vi "PPS_TRAJECTORY_CMD_FOLLOW_SWERVE.vi"(6 "Pass_Through_Time":dbl=-1.0 format="%33.4f", 8 "Init":bool) -> (0 "AtReference":bool, 1 "Complete":bool, 3 "Chassis Velocity Target SI":T1 {"vOmega" format="%10.3f"; "vY" format="%10.3f"; "vX" format="%10.3f"})   [LabVIEW 2019]
uses:
  <vilib>/Rock Robotics/WPI/ThirdParty/JAS_Junk/TrajLib/TypeDef/CHASSIS_SPEEDS.ctl
  <vilib>/Rock Robotics/WPI/ThirdParty/JAS_Junk/TrajLib/VI/Util_GetTime_U32.vi
  <vilib>/Rock Robotics/WPI/ThirdParty/JAS_Junk/TrajLib/ProfiledPIDController_NewPeriod.vi
  <vilib>/Rock Robotics/WPI/ThirdParty/JAS_Junk/TrajLib/ProfiledPIDController_SetIntegratorRange.vi
  <vilib>/Rock Robotics/WPI/ThirdParty/JAS_Junk/TrajLib/ProfiledPIDController_DisableContInput.vi
  <vilib>/Rock Robotics/WPI/ThirdParty/JAS_Junk/TrajLib/ProfiledPIDController_EnableContInput.vi
  <vilib>/Rock Robotics/WPI/ThirdParty/JAS_Junk/TrajLib/TrapProfConstraint_New.vi
  <vilib>/Rock Robotics/WPI/ThirdParty/JAS_Junk/TrajLib/Pose2d_New.vi
  <vilib>/Rock Robotics/WPI/ThirdParty/JAS_Junk/TrajLib/Conv_Deg_Radians.vi
  <vilib>/Rock Robotics/WPI/ThirdParty/JAS_Junk/TrajLib/TrapProfState_New.vi
  <vilib>/Rock Robotics/WPI/ThirdParty/JAS_Junk/TrajLib/PIDController_NewPeriod.vi
  <vilib>/Rock Robotics/SystemInterfaces/NetworkCommunication/NetComm_UsageReport_report.vi
  <vilib>/Rock Robotics/WPI/ThirdParty/JAS_Junk/TrajLib/PIDController_SetIntegratorRange.vi
  <vilib>/Rock Robotics/WPI/ThirdParty/JAS_Junk/TrajLib/PIDController_DisableContinousInput.vi
  <vilib>/Rock Robotics/WPI/ThirdParty/JAS_Junk/TrajLib/PIDController_EnableContinousInput.vi
  <vilib>/Rock Robotics/WPI/ThirdParty/JAS_Junk/TrajLib/Rotation2d_CreateAngle.vi
  <vilib>/Rock Robotics/WPI/ThirdParty/JAS_Junk/TrajLib/Translation2d_Create.vi
  PPS_TRAJECTORY_GLOBALS.vi
  Swerve_Drive_System/PPS_DRIVE_GLOBALS.vi
  <vilib>/Rock Robotics/WPI/ThirdParty/JAS_Junk/TrajLib/Globals/Util_LibraryGlobals.vi
  <vilib>/Rock Robotics/WPI/ThirdParty/JAS_Junk/TrajLib/VI/Util_GetTime_U64.vi
  <vilib>/Rock Robotics/WPI/ThirdParty/JAS_Junk/TrajLib/Trajectory_Library.lvlib
  <vilib>/Rock Robotics/WPI/ThirdParty/MJansen/PathPlanner/PathPlanner24.lvlib
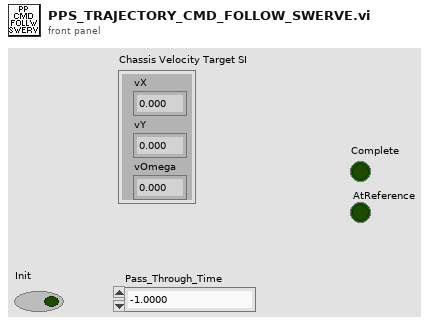
[diagram p1: front panel]
types:
  T1 = typedef "Trajectory_Library.lvlib/CHASSIS_SPEEDS.ctl" = cluster{"vX":dbl, "vY":dbl, "vOmega":dbl}
  T2 = typedef "PathPlanner24.lvlib/PathPlannerPath.ctl" = cluster{"BezierPoints":T3[], "PreviewStartingRotation":T4, "Reversed":bool, "RotationTargets":T5[], "ConstraintZones":T6[], "EventMarkers":T8[], "GlobalConstraints":T7, "GoalEndState":T11, "AllPoints":T12[]}
  T3 = typedef "Trajectory_Library.lvlib/TRANSLATION2D.ctl" = cluster{"X":dbl, "Y":dbl}
  T4 = typedef "Trajectory_Library.lvlib/ROTATION2D.ctl" = cluster{"VALUE":dbl, "COS":dbl, "SIN":dbl}
  T5 = typedef "PathPlanner24.lvlib/PathPlannerRotationTarget.ctl" = cluster{"target":T4, "WaypointRelativePosition":dbl, "Exists":bool}
  T6 = typedef "PathPlanner24.lvlib/PathPlannerConstraintsZone.ctl" = cluster{"minWaypointPos":dbl, "maxWaypointPos":dbl, "Constraints":T7, "Present":bool}
  T7 = typedef "PathPlanner24.lvlib/PathPlannerPathConstraints.ctl" = cluster{"MaxVelocityMps;":dbl, "MaxAccelerationMpsSq;":dbl, "MaxAngularVelRadPsEc;":dbl, "MaxAngularAccRadPSecSq":dbl, "Exists":bool}
  T8 = typedef "PathPlanner24.lvlib/PathPlannerEventMarker.ctl" = cluster{"WaypointRelativePos":dbl, "minimumTriggerDistance":dbl, "markerPos":T3, "lastRobotPos":T3, "Command":T9, "markerPos Exists":bool, "LastRobotPoseExists":bool, "Triggered":bool}
  T9 = typedef "PathPlanner24.lvlib/PathPlannerCommandUtil.ctl" = cluster{"waitTime":dbl, "name":string, "pathName":string, "commands":cluster{"type":T10, "waitTime":dbl, "name":string, "pathName":string}[], "type":T10}
  T10 = typedef "PathPlanner24.lvlib/PathPlanner_CommandUtilType_ENUM.ctl" = enum16{"Unknown", "Wait", "Named", "Path", "Sequential", "Parallel", "Race", "Deadline"}
  T11 = typedef "PathPlanner24.lvlib/PathPlannerGoalEndState.ctl" = cluster{"Velocity":dbl, "Rotation":T4}
  T12 = typedef "PathPlanner24.lvlib/PathPlannerPathPoint.ctl" = cluster{"Position":T3, "HolonomicRotation":T4, "DistAlongPath":dbl, "CurveRadius":dbl, "MaxV":dbl, "Constraints":T7, "HolonomicRotationExists":bool}
  T13 = typedef "Trajectory_Library.lvlib/PID_TUNING.ctl" = cluster{"Kp":dbl, "Ki":dbl, "Kd":dbl, "MaximumIntegral":dbl, "MinimumIntegral":dbl}
  T14 = typedef "Trajectory_Library.lvlib/POSE2D.ctl" = cluster{"TRANSLATION":T3, "ROTATION":T4}
  T15 = typedef "Trajectory_Library.lvlib/PROFILED_PID_CONTROLLER.ctl" = cluster{"Controller":T16, "Goal":T17, "Setpoint":T17, "Constraint":T18}
  T16 = typedef "Trajectory_Library.lvlib/PID_CONTROLLER.ctl" = cluster{"Kp":dbl, "Ki":dbl, "Kd":dbl, "Period":dbl, "Max_Integral":dbl, "Min_Integral":dbl, "Max_Input":dbl, "Min_Input":dbl, "Continuous":bool, "PositionError":dbl, "VelocityError":dbl, "PrevError":dbl, "TotalError":dbl, "PositionTolerance":dbl, "VelocityTolerance":dbl, "SetPoint":dbl, "Kf":dbl, "Prev_Deriv":dbl, "Prev_Deriv 2":dbl, "DerivativeFilter":bool, "Min_Output":dbl, "Max_Output":dbl, "Prev_F_P":dbl, "Prev_F_P_2":dbl, "AntiWindupActive":bool, "Measurement":dbl}
  T17 = typedef "Trajectory_Library.lvlib/TRAPEZOID_PROFILE_STATE.ctl" = cluster{"Position":dbl, "Velocity":dbl}
  T18 = typedef "Trajectory_Library.lvlib/TRAPEZOID_PROFILE_CONSTRAINT.ctl" = cluster{"MaxVelocity":dbl, "MaxAcceleration":dbl}
  T19 = typedef "PathPlanner24.lvlib/PathPlannerReplanningConfig.ctl" = cluster{"enableInitialReplanning":bool, "enableDynamicReplanning":bool, "dynamicReplanningTotalErrorThreshold":dbl, "dynamicReplanningErrorSpikeThreshold":dbl}
  T20 = typedef "Trajectory_Library.lvlib/HOLONOMIC_PACK_TUNING.ctl" = cluster{"X PID Tuning":T13, "Y PID Tuning":T13, "thetaProfiledPID_CTRL":T15}
  T21 = typedef "PathPlanner24.lvlib/PathPlannerCmdFollowHolConfig.ctl" = cluster{"HOLONOMIC_CTRL_PACK_TUNING":T20, "Max Wheel Speed M/S":dbl, "Tolerance SI":T14, "Drive Base Radius M":dbl, "ControlPastEnd_Sec":dbl, "ReplanningConfig":T19, "Period_Sec":dbl, "Trigger Events":bool}
  T22 = typedef "Trajectory_Library.lvlib/HOLONOMIC_DRV_CTRL.ctl" = cluster{"poseTolerance":T14, "poseError":T14, "Enabled":bool, "PID_xCtrl":T16, "PID_yCtrl":T16, "PROF_PID_thetaCtrl":T15, "RotationError":T4, "FirstRun":bool}
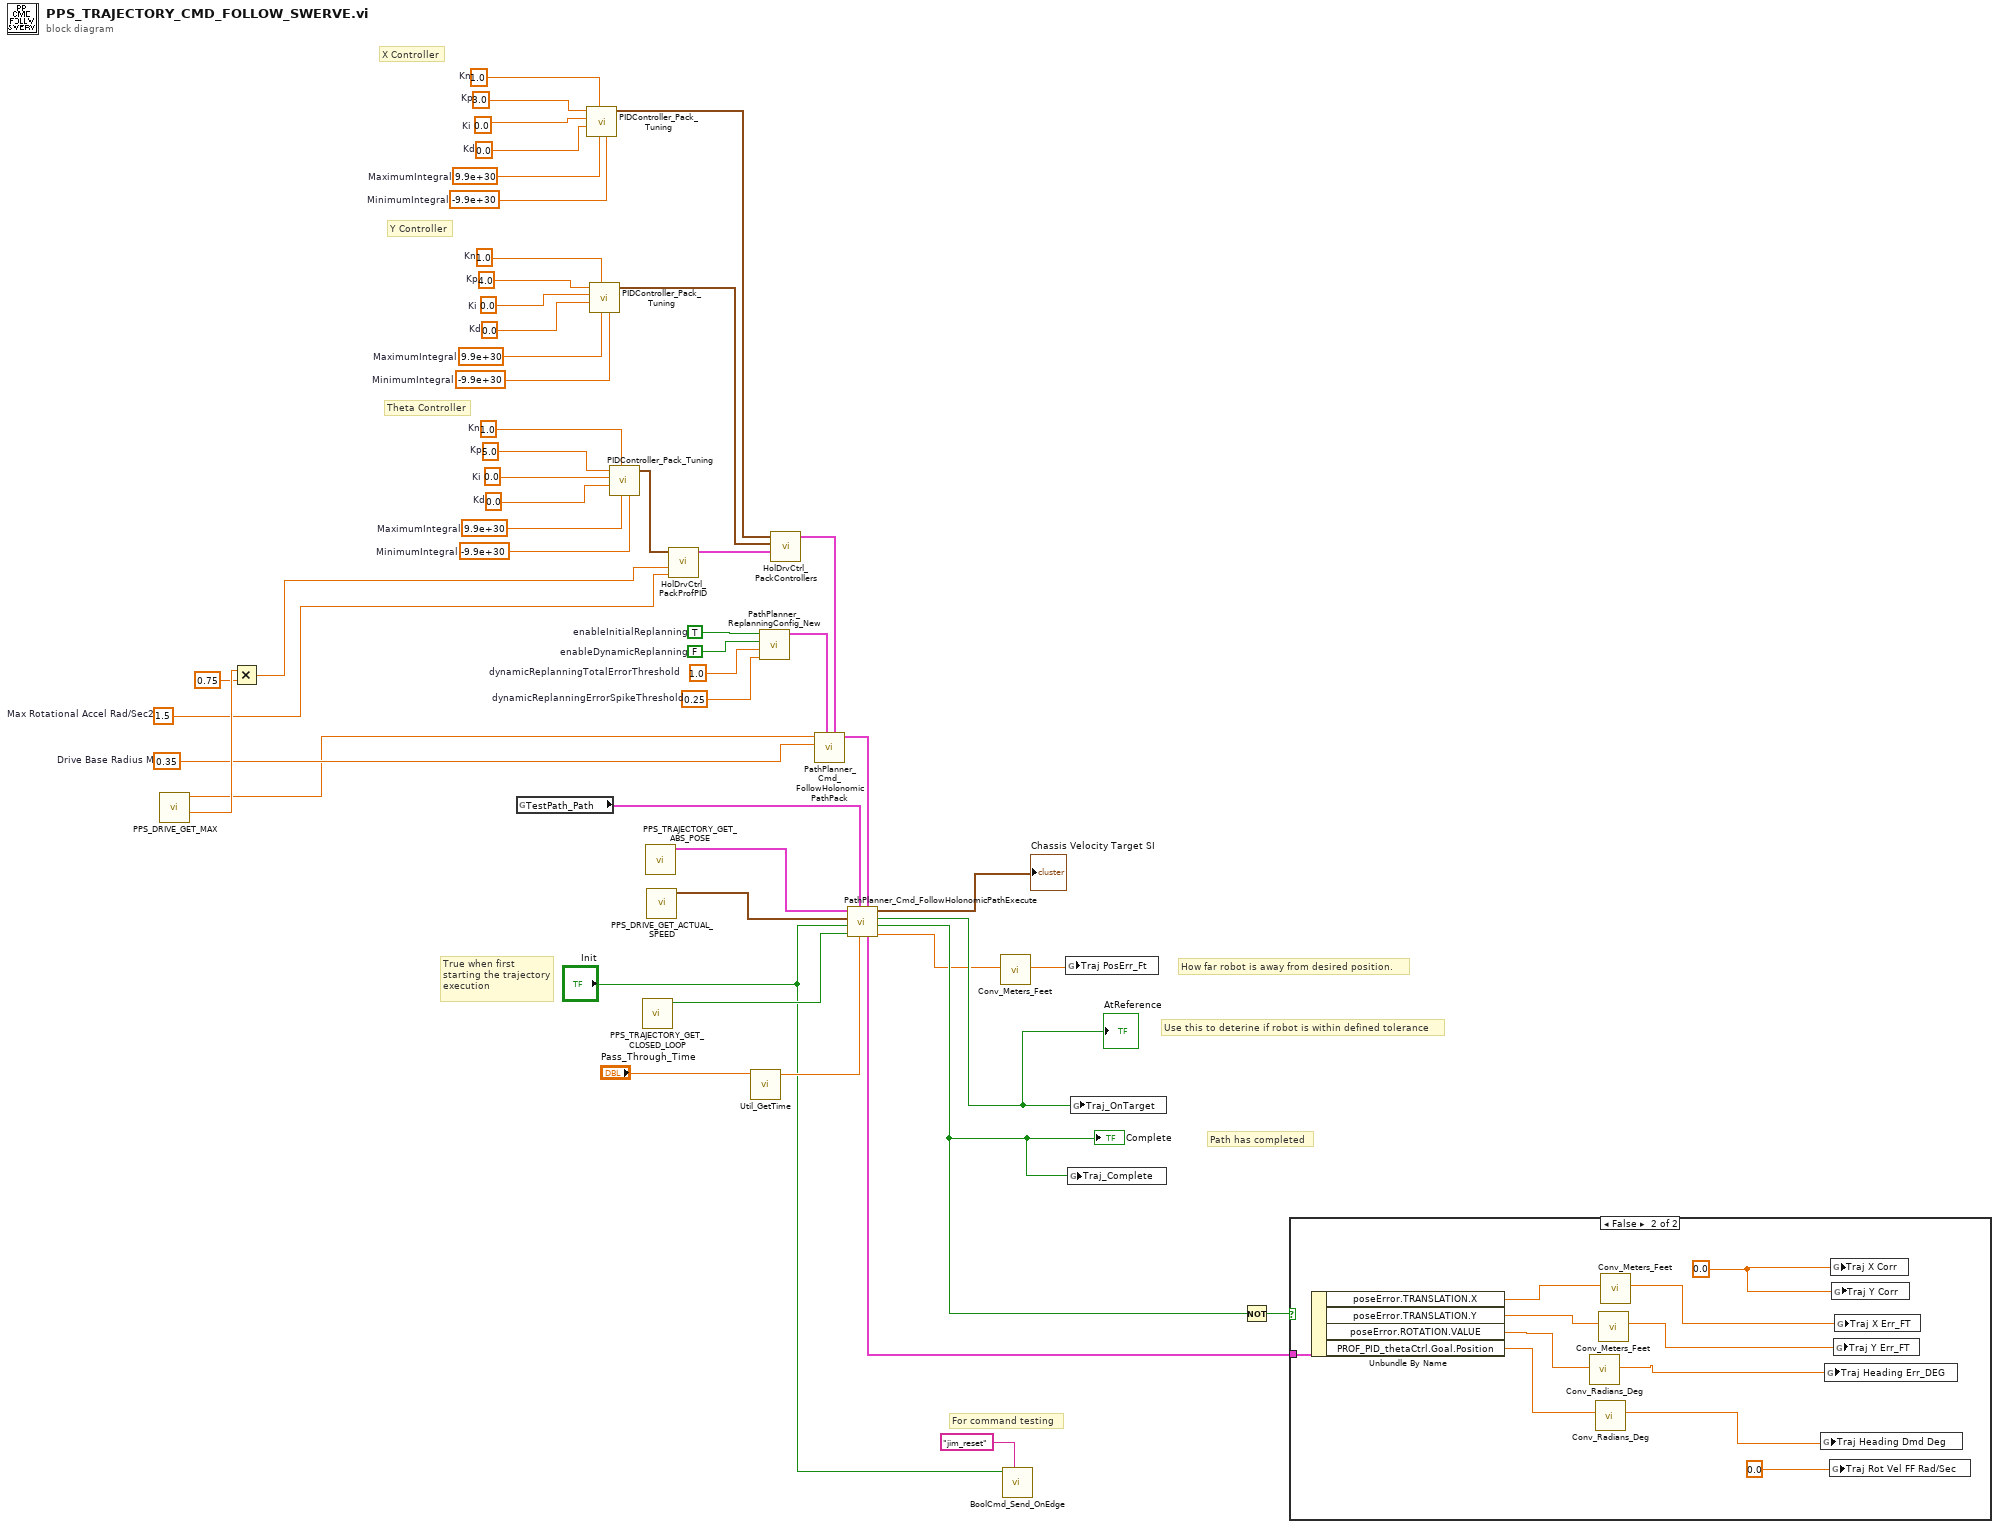
[diagram p0: block diagram]
diagram:
  w48 = TRUE  # enableInitialReplanning
  w47 = FALSE  # enableDynamicReplanning
  w46 = 1.0  # dynamicReplanningTotalErrorThreshold
  w45 = 0.25  # dynamicReplanningErrorSpikeThreshold
  w35 = 1.0  # Kn
  w32 = 5.0  # Kp
  w23 = 0.0  # Ki
  w22 = 0.0  # Kd
  w21 = 9.9e+30  # MaximumIntegral
  w20 = -9.9e+30  # MinimumIntegral
  w37 = 1.0  # Kn
  w34 = 3.0  # Kp
  w31 = 0.0  # Ki
  w30 = 0.0  # Kd
  w29 = 9.9e+30  # MaximumIntegral
  w28 = -9.9e+30  # MinimumIntegral
  w36 = 1.0  # Kn
  w33 = 4.0  # Kp
  w27 = 0.0  # Ki
  w26 = 0.0  # Kd
  w25 = 9.9e+30  # MaximumIntegral
  w24 = -9.9e+30  # MinimumIntegral
  w17 = 0.35  # Drive Base Radius M
  w18 = 1.5  # Max Rotational Accel Rad/Sec2
  # "For command testing"
  # "Path has completed"
  # "How far robot is away from desired position."
  # "Use this to deterine if robot is within defined tolerance"
  # "Theta Controller"
  # "Y Controller"
  # "X Controller"
  # "True when first\nstarting the trajectory\nexecution"
  n1 = call "PPS_DRIVE_GET_MAX.vi"() -> ("Max Rotational Vel (Rad/Sec)"=w50:dbl, "Max Wheel Vel (Meter/Sec)"=w11:dbl)  [unwired: 10 in]
  n2 = Multiply(x=w50, y=0.75) -> (x*y=w19:dbl)
  n3 = global read "PPS_TRAJECTORY_GLOBALS.vi" "TestPath_Path"() -> (w16:T2)
  n4 = call <vilib>:"PIDController_Pack_Tuning.vi"("MinimumIntegral"=w28, "MaximumIntegral"=w29, "Kn"=w37, "Kd"=w30, "Ki"=w31, "Kp"=w34) -> ("PID Tuning"=w41:T13)  [unwired: 5 in]
  n5 = call <vilib>:"PIDController_Pack_Tuning.vi"("MinimumIntegral"=w24, "MaximumIntegral"=w25, "Kn"=w36, "Kd"=w26, "Ki"=w27, "Kp"=w33) -> ("PID Tuning"=w42:T13)  [unwired: 5 in]
  n6 = call <vilib>:"PIDController_Pack_Tuning.vi"("MinimumIntegral"=w20, "MaximumIntegral"=w21, "Kn"=w35, "Kd"=w22, "Ki"=w23, "Kp"=w32) -> ("PID Tuning"=w38:T13)  [unwired: 5 in]
  n7 = call "PPS_TRAJECTORY_GET_CLOSED_LOOP.vi"() -> ("AUTO_CLOSED_LOOP"=w13:bool)  [unwired: 11 in]
  n8 = call "PPS_TRAJECTORY_GET_ABS_POSE.vi"() -> ("Absolute Odometry Pose"=w15:T14)  [unwired: 11 in]
  n9 = call "PPS_DRIVE_GET_ACTUAL_SPEED.vi"() -> ("Drv Chassis Actual Velocity"=w14:T1)  [unwired: 11 in]
  n10 = call <vilib>:"HolDrvCtrl_PackProfPID.vi"("Max Accel"=w18, "Max Speed"=w19, "Theta PID Tuning"=w38) -> ("Theta PID CONTROLLER"=w43:T15)  [unwired: 8 in]
  n11 = call <vilib>:"Util_GetTime.vi"("Pass_Through_Time"="Pass_Through_Time") -> ("FPGA_Time_Seconds"=w10:dbl)  [unwired: 8 in, 2 out]
  n12 = call <vilib>:"PathPlanner_ReplanningConfig_New.vi"("dynamicReplanningErrorSpikeThreshold"=w45, "dynamicReplanningTotalErrorThreshold"=w46, "enableDynamicReplanning"=w47, "enableInitialReplanning"=w48) -> ("ReplanningConfig"=w44:T19)  [unwired: 7 in]
  n13 = call <vilib>:"HolDrvCtrl_PackControllers.vi"("thetaProfiledPID_CTRL"=w43, "Y PID Tuning"=w42, "X PID Tuning"=w41) -> ("HOLONOMIC_CTRL_PACK_TUNING"=w40:T20)  [unwired: 8 in]
  n14 = call <vilib>:"PathPlanner_Cmd_FollowHolonomicPathPack.vi"("HOLONOMIC_CTRL_PACK_TUNING"=w40, "ReplanningConfig"=w44, "Drive Base Radius M"=w17, "Max Wheel Speed M/S"=w11) -> ("PathPlanner_Ctrl_HolDrvConfig"=w39:T21)  [unwired: 7 in]
  n15 = call <vilib>:"PathPlanner_Cmd_FollowHolonomicPathExecute.vi"("PathPlanner_Cmd_FollowHolConfig"=w39, "PassthroughTime_SEC"=w10, "PathPlannerPath"=w16, "Enabled"=w13, "Reset"="Init", "CurrentChassisSpeeds"=w14, "Current Pose SI"=w15) -> ("Position Error M"=w3:dbl, "Complete"=w5:bool, "At Reference"=w7:bool, "calcChassisSpeed"=→"Chassis Velocity Target SI":T1, "outHOLONOMIC_DRV_CTRL"=w8:T22)
  "AtReference" <- w7
  "Complete" <- w5
  n16 = call <vilib>:"Conv_Meters_Feet.vi"("Meters"=w3) -> ("Feet"=w4:dbl)  [unwired: 10 in]
  n17 = call <vilib>:"BoolCmd_Send_OnEdge.vi"("Command Name"="jim_reset", "Value"="Init") -> ()  [unwired: 9 in, 1 out]
  n18 = global write "PPS_TRAJECTORY_GLOBALS.vi" "Traj PosErr_Ft"(w4) -> ()
  n19 = global write "PPS_TRAJECTORY_GLOBALS.vi" "Traj_Complete"(w5) -> ()
  n20 = global write "PPS_TRAJECTORY_GLOBALS.vi" "Traj_OnTarget"(w7) -> ()
  n21 = Not(x=w5) -> (.not. x?=w6:bool)
  n22 = case shown="False" w6 {
    tunnel: w8 -> [_ w57]
    frame True {
    }
    frame False {
      w61 = 0.0 ("Y Corr")
      n23 = Unbundle By Name(w57) -> ("poseError.TRANSLATION.X"=w56:dbl, "poseError.TRANSLATION.Y"=w55:dbl, "poseError.ROTATION.VALUE"=w54:dbl, "PROF_PID_thetaCtrl.Goal.Position"=w52:dbl)
      n24 = call <vilib>:"Conv_Radians_Deg.vi"("Radians"=w54) -> ("Degrees"=w53:dbl)  [unwired: 10 in]
      n25 = call <vilib>:"Conv_Radians_Deg.vi"("Radians"=w52) -> ("Degrees"=w51:dbl)  [unwired: 10 in]
      n26 = call <vilib>:"Conv_Meters_Feet.vi"("Meters"=w55) -> ("Feet"=w60:dbl)  [unwired: 10 in]
      n27 = call <vilib>:"Conv_Meters_Feet.vi"("Meters"=w56) -> ("Feet"=w59:dbl)  [unwired: 10 in]
      n28 = global write "PPS_TRAJECTORY_GLOBALS.vi" "Traj Heading Dmd Deg"(w51) -> ()
      n29 = global write "PPS_TRAJECTORY_GLOBALS.vi" "Traj Heading Err_DEG"(w53) -> ()
      n30 = global write "PPS_TRAJECTORY_GLOBALS.vi" "Traj Rot Vel FF Rad/Sec"(0.0 ("Traj Heading Dmd Deg")) -> ()
      n31 = global write "PPS_TRAJECTORY_GLOBALS.vi" "Traj X Corr"(w61) -> ()
      n32 = global write "PPS_TRAJECTORY_GLOBALS.vi" "Traj Y Corr"(w61) -> ()
      n33 = global write "PPS_TRAJECTORY_GLOBALS.vi" "Traj Y Err_FT"(w60) -> ()
      n34 = global write "PPS_TRAJECTORY_GLOBALS.vi" "Traj X Err_FT"(w59) -> ()
    }
  }
